vi "FTW-Collection-ToKeyValuePairs.vi"(0 "Collection":refnum<class "FTW-Collection.lvclass">, 11 "error in":errorcluster) -> (4 "Collection out":refnum<class "FTW-Collection.lvclass">, 6 "Key-Value Pairs":T1[](array[typedef]), 15 "error out":errorcluster)   [LabVIEW 2013, in "FTW-Collection.lvclass"]
uses:
  FTW-Collection.lvclass
  FTW-Collection-KeyValuePair.ctl
panel:
  # "Inputs"
  # "Outputs"
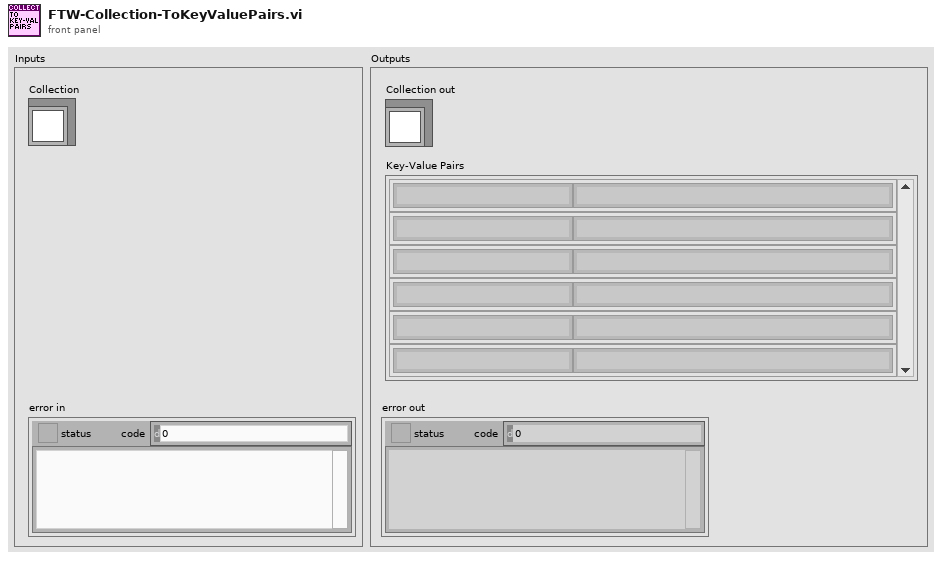
[diagram p1: front panel]
types:
  T1 = typedef "FTW-Collection-KeyValuePair.ctl" = cluster{"Key":string, "Value":string}
  T2 = typedef "FTW-Collection-KeyVariantPair.ctl" = cluster{"Key":string, "Value":variant}
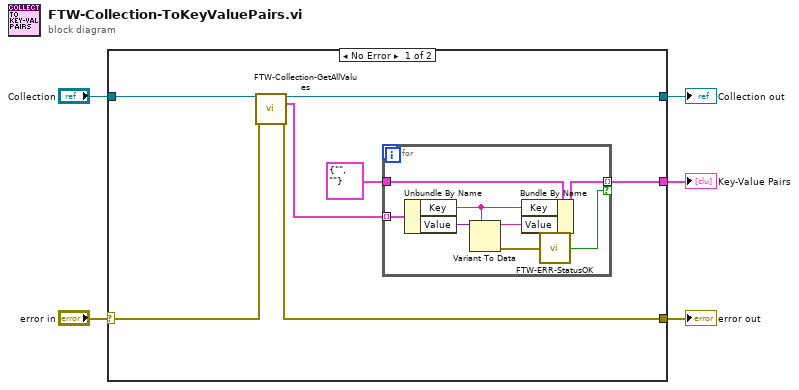
[diagram p0: block diagram]
diagram:
  n1 = case shown="No Error" "error in" {
    selector: "error in" -> [w8 w22]
    tunnel: [w7 w22] -> w5
    tunnel: [w9 w21] -> w3
    tunnel: "Collection" -> [w10 w21]
    tunnel: [w11 _] -> w1
    frame No Error {
      n2 = call "FTW-Collection-GetAllValues.vi"("Collection"=w10, "error in"=w8) -> ("Collection out"=w9:refnum<class "FTW-Collection.lvclass">, "Key-Variant Pairs"=w6:T2[], "error out"=w7:errorcluster)  [unwired: 11 in]
      n3 = for {
        tunnel: [w17] -> w11 mode=indexing if=w19
        tunnel: T1 {"Key"="", "Value"=""} ("Key-Value Pair") -> [w18]
        tunnel: w6 -> [w15] mode=indexing
        n4 = Unbundle By Name(w15) -> ("Key"=w14:string, "Value"=w13:variant)
        n5 = Variant To Data(type=w14, Variant=w13) -> (data=w16:string, error out=w20:errorcluster)  [unwired: 1 in]
        n6 = Bundle By Name(cluster=w18, "Key"=w14, "Value"=w16) -> (w17:T1)
        n7 = call "FTW-ERR-StatusOK.vi"("error to check"=w20) -> ("Status OK?"=w19:bool)
      }
    }
    frame Error {
    }
  }
  "error out" <- w5
  "Collection out" <- w3
  "Key-Value Pairs" <- w1
